vi "ZDataVIS_Unflatten.vi"(5 "diff points":dbl, 7 "sampling info":T2={"# Vslow"=1, "# Vfast"=1, "# Vslowest"=1, "# Samples per IV"=1}, 8 "error in (no error)":errorcluster, 9 "Vfast":dbl[](array[numeric]), 10 "Vsd":dbl[](array[numeric]), 11 "I":dbl[](array[numeric])) -> (0 "error out":errorcluster, 1 "Vfast":dbl[][](array[numeric]), 3 "DVR ready":T1(array[cluster]))   [LabVIEW 2016]
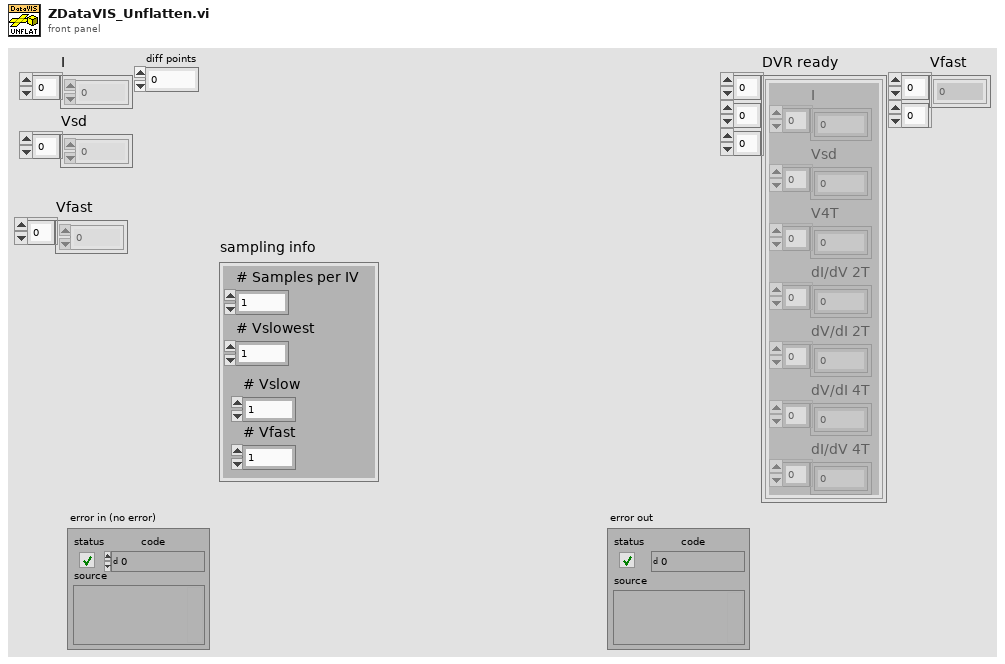
[diagram p1: front panel]
types:
  T1 = cluster{"I":dbl[], "Vsd":dbl[], "V4T":dbl[], "dI/dV 2T":dbl[], "dV/dI 2T":dbl[], "dV/dI 4T":dbl[], "dI/dV 4T":dbl[]}[][][]
  T2 = cluster{"# Vslow":i32, "# Vfast":i32, "# Vslowest":i32, "# Samples per IV":i32}
  T3 = cluster{"I":dbl[], "Vsd":dbl[], "V4T":dbl[], "dI/dV 2T":dbl[], "dV/dI 2T":dbl[], "dV/dI 4T":dbl[], "dI/dV 4T":dbl[]}
  T4 = cluster{"Decimated Array":dbl[], "Decimated Array":dbl[]}
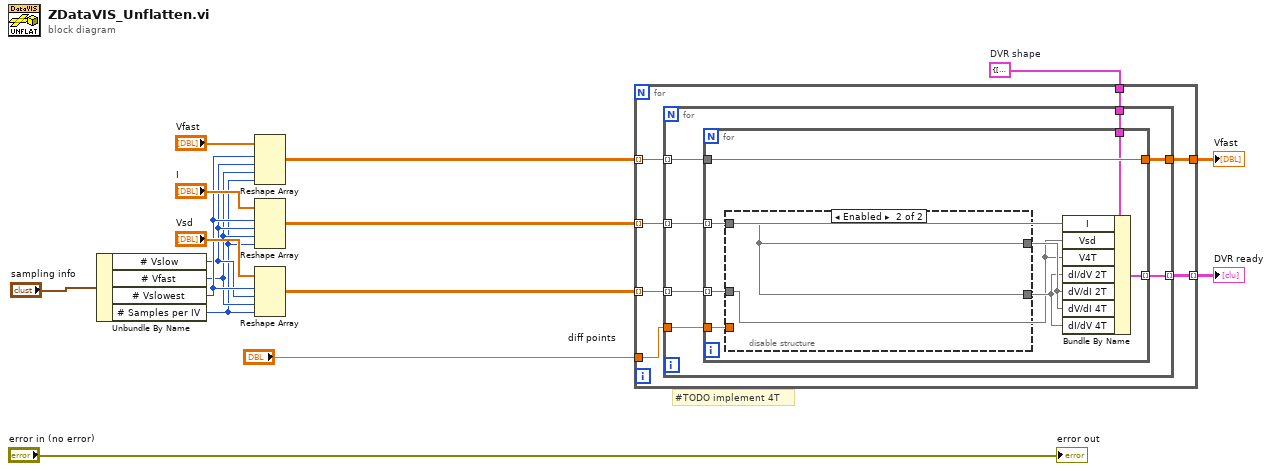
[diagram p0: block diagram]
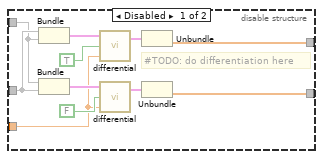
[diagram p2: hidden frame]
diagram:
  w1 = T3 {"I"=[], "Vsd"=[], "V4T"=[], "dI/dV 2T"=[], "dV/dI 2T"=[], "dV/dI 4T"=[], "dI/dV 4T"=[]}  # DVR shape
  # "#TODO implement 4T"
  n1 = Unbundle By Name("sampling info") -> ("# Vslow"=w8:i32, "# Vfast"=w7:i32, "# Vslowest"=w9:i32, "# Samples per IV"=w6:i32)
  n2 = Reshape Array("Vfast", w9, w8, w7, w6) -> (w3:dbl[][][][])
  n3 = Reshape Array("I", w9, w8, w7, w6) -> (w13:dbl[][][][])
  n4 = Reshape Array("Vsd", w9, w8, w7, w6) -> (w5:dbl[][][][])
  n5 = for {
    tunnel: [w23] -> w12 mode=indexing
    tunnel: w13 -> [w22] mode=indexing
    tunnel: w5 -> [w21] mode=indexing
    tunnel: w3 -> [w20] mode=indexing
    tunnel: [w19] -> w4
    tunnel: "diff points" -> [w18]
    tunnel: w1 -> [w17]
    n6 = for {
      tunnel: [w30] -> w23 mode=indexing
      tunnel: w22 -> [w29] mode=indexing
      tunnel: w21 -> [w28] mode=indexing
      tunnel: w20 -> [w27] mode=indexing
      tunnel: [w26] -> w19
      tunnel: w18 -> [w25]
      tunnel: w17 -> [w24]
      n7 = for {
        tunnel: [w38] -> w30 mode=indexing
        tunnel: w29 -> [w32] mode=indexing
        tunnel: w28 -> [w33] mode=indexing
        tunnel: w27 -> [w37]
        tunnel: [w37] -> w26
        tunnel: w25 -> [w36]
        tunnel: w24 -> [w31]
        n8 = disable-structure shown="Enabled" {
          disable-tunnel: w36 -> [w45 _]
          disable-tunnel: [w42 w50] -> w35
          disable-tunnel: [w41 w50] -> w34
          disable-tunnel: w33 -> [w40 _]
          disable-tunnel: w32 -> [w39 w50]
          frame Disabled {
            # "#TODO: do differentiation here"
            n9 = Bundle("Vsd"=w40, "I"=w39) -> (w46:cluster{"Vsd":dbl[], "I":dbl[]})  [unwired: 1 in]
            n10 = Bundle("I"=w39, "Vsd"=w40) -> (w49:cluster{"I":dbl[], "Vsd":dbl[]})  [unwired: 1 in]
            n11 = call <userlib>:"differential.vi"("Numeric"=w45, "dy/dx vs x"=TRUE, "A vs B 2"=w46) -> ("A vs B 3"=w43:T4)  [unwired: 1 in]
            n12 = call <userlib>:"differential.vi"("Numeric"=w45, "dy/dx vs x"=FALSE, "A vs B 2"=w49) -> ("A vs B 3"=w47:T4)  [unwired: 1 in]
            n13 = Unbundle(w43) -> ("Decimated Array"=w42:dbl[])  [unwired: 1 out]
            n14 = Unbundle(w47) -> ("Decimated Array"=w41:dbl[])  [unwired: 1 out]
          }
          frame Enabled {
          }
        }
        n15 = Bundle By Name(cluster=w31, "I"=w32, "Vsd"=w33, "V4T"=w33, "dI/dV 2T"=w34, "dV/dI 2T"=w35, "dV/dI 4T"=w35, "dI/dV 4T"=w34) -> (w38:T3)
      }
    }
  }
  "DVR ready" <- w12
  "Vfast" <- w4
  "error out" <- "error in (no error)"
